vi "curr_measurement.vi"() -> ()   [LabVIEW 2018]
uses:
  <vilib>/Utility/file.llb/Write Delimited Spreadsheet (string).vi
  <instrlib>/Keithley 648X Series/Keithley 648X Series.lvlib
  <vilib>/Analysis/NI_AALBase.lvlib
panel:
  in  "Range (nA)":u16(ring)=6 items=["20mA", "2mA", "200uA", "20uA", "2uA", "200nA", "20nA", "2nA"]
  out "Waveform Graph":dbl[](graph)=[-9.351637e-09, -9.150208e-09, -1.001427e-08, -8.748215e-09, -8.522931e-09, -8.492725e-09, -9.785064e-09, -9.437517e-09, -9.272836e-09, -9.83262e-09, -9.335976e-09, -9.824586e-09, -9.370058e-09, -9.594313e-09, -9.258558e-09, -1.001164e-08, -9.479965e-09, -9.818684e-09, -8.33904e-09, -1.000336e-08, -9.407453e-09, -9.480965e-09, -9.881598e-09, -9.252624e-09, -9.527317e-09, -9.713401e-09, -8.709614e-09, -1.017135e-08, -9.863273e-09, -9.304885e-09, -1.037396e-08, -8.691322e-09, -9.202171e-09, -9.427193e-09, -9.452378e-09, -9.301955e-09, -9.93608e-09, -1.016247e-08, -9.657593e-09, -9.639637e-09, -9.532354e-09, -9.976174e-09, -9.564596e-09, -9.419945e-09, -9.793799e-09, -9.572672e-09, -9.966555e-09, -9.634946e-09, -9.932353e-09, -9.015443e-09, -9.172623e-09, -9.54698e-09, -9.282637e-09, -9.429553e-09, -1.039608e-08, -9.177771e-09, -9.569834e-09, -9.949303e-09, -9.517366e-09, -9.941039e-09, -9.143115e-09, -9.300412e-09, -9.838465e-09, -1.04458e-08, -8.665026e-09, -1.010992e-08, -9.321636e-09, -9.305311e-09, -9.199045e-09, -9.379991e-09, -1.014202e-08, -9.659195e-09, -1.016863e-08, -8.558392e-09, -8.893284e-09, -9.430091e-09, -1.035581e-08, -8.855966e-09, -9.206192e-09, -9.404848e-09, -9.820688e-09, -9.750344e-09, -9.513444e-09, -9.751563e-09, -1.025721e-08, -9.897644e-09, -9.474945e-09, -9.120714e-09, -9.959159e-09, -9.044635e-09, -9.964291e-09, -9.179353e-09, -9.380761e-09, -9.697832e-09, -9.19995e-09, -9.515208e-09, -9.913225e-09, -9.952196e-09, -9.35025e-09, -9.10259e-09, -9.434953e-09]
  out "Current Error":dbl=4.475602666243125e-11
  out "Current Mean":dbl=-9.525059320000003e-09 format="%e"
  out "Measurements":dbl[](array[numeric])=[-9.150208e-09, -1.001427e-08, -8.748215e-09, -8.522931e-09, -8.492725e-09, -9.785064e-09, -9.437517e-09, -9.272836e-09, -9.83262e-09, -9.335976e-09, -9.824586e-09, -9.370058e-09, -9.594313e-09, -9.258558e-09, -1.001164e-08, -9.479965e-09, -9.818684e-09, -8.33904e-09, -1.000336e-08, -9.407453e-09, -9.480965e-09, -9.881598e-09, -9.252624e-09, -9.527317e-09, -9.713401e-09, -8.709614e-09, -1.017135e-08, -9.863273e-09, -9.304885e-09, -1.037396e-08, -8.691322e-09, -9.202171e-09, -9.427193e-09, -9.452378e-09, -9.301955e-09, -9.93608e-09, -1.016247e-08, -9.657593e-09, -9.639637e-09, -9.532354e-09, -9.976174e-09, -9.564596e-09, -9.419945e-09, -9.793799e-09, -9.572672e-09, -9.966555e-09, -9.634946e-09, -9.932353e-09, -9.015443e-09, -9.172623e-09, -9.54698e-09, -9.282637e-09, -9.429553e-09, -1.039608e-08, -9.177771e-09, -9.569834e-09, -9.949303e-09, -9.517366e-09, -9.941039e-09, -9.143115e-09, -9.300412e-09, -9.838465e-09, -1.04458e-08, -8.665026e-09, -1.010992e-08, -9.321636e-09, -9.305311e-09, -9.199045e-09, -9.379991e-09, -1.014202e-08, -9.659195e-09, -1.016863e-08, -8.558392e-09, -8.893284e-09, -9.430091e-09, -1.035581e-08, -8.855966e-09, -9.206192e-09, -9.404848e-09, -9.820688e-09, -9.750344e-09, -9.513444e-09, -9.751563e-09, -1.025721e-08, -9.897644e-09, -9.474945e-09, -9.120714e-09, -9.959159e-09, -9.044635e-09, -9.964291e-09, -9.179353e-09, -9.380761e-09, -9.697832e-09, -9.19995e-09, -9.515208e-09, -9.913225e-09, -9.952196e-09, -9.35025e-09, -9.10259e-09, -9.434953e-09]
  out "error out":T1
  in  "Insert Voltage;Divider Current":string="3498.5;714.27"
  out "Stop Time string":string="20/02/2023 10:43:20"
  in  "file path (dialog if empty)":path=path "C:/Users/david/cernbox/Work/Detectors-Characterizations/monitoringGEM/P5_measurements/20022023/20022023.csv"
  out "Format Data":string[](array[string])=["Start time:", "Stop time:", "Voltage/Divider Current:", "Mean Anodic Current(A):", "Gaussian Error(A):"]
  out "Start time string":string="20/02/2023 10:42:43,00"
  in  "Interactions+1":i32=101
  out "Last measurement":dbl=-9.434953e-09
  in  "Autorange (T: Enable)":bool
  in  "error in (no error)":errorcluster
  in  "VISA resource name":refnum<visa-resource-name>="GPIB0::22::INSTR"
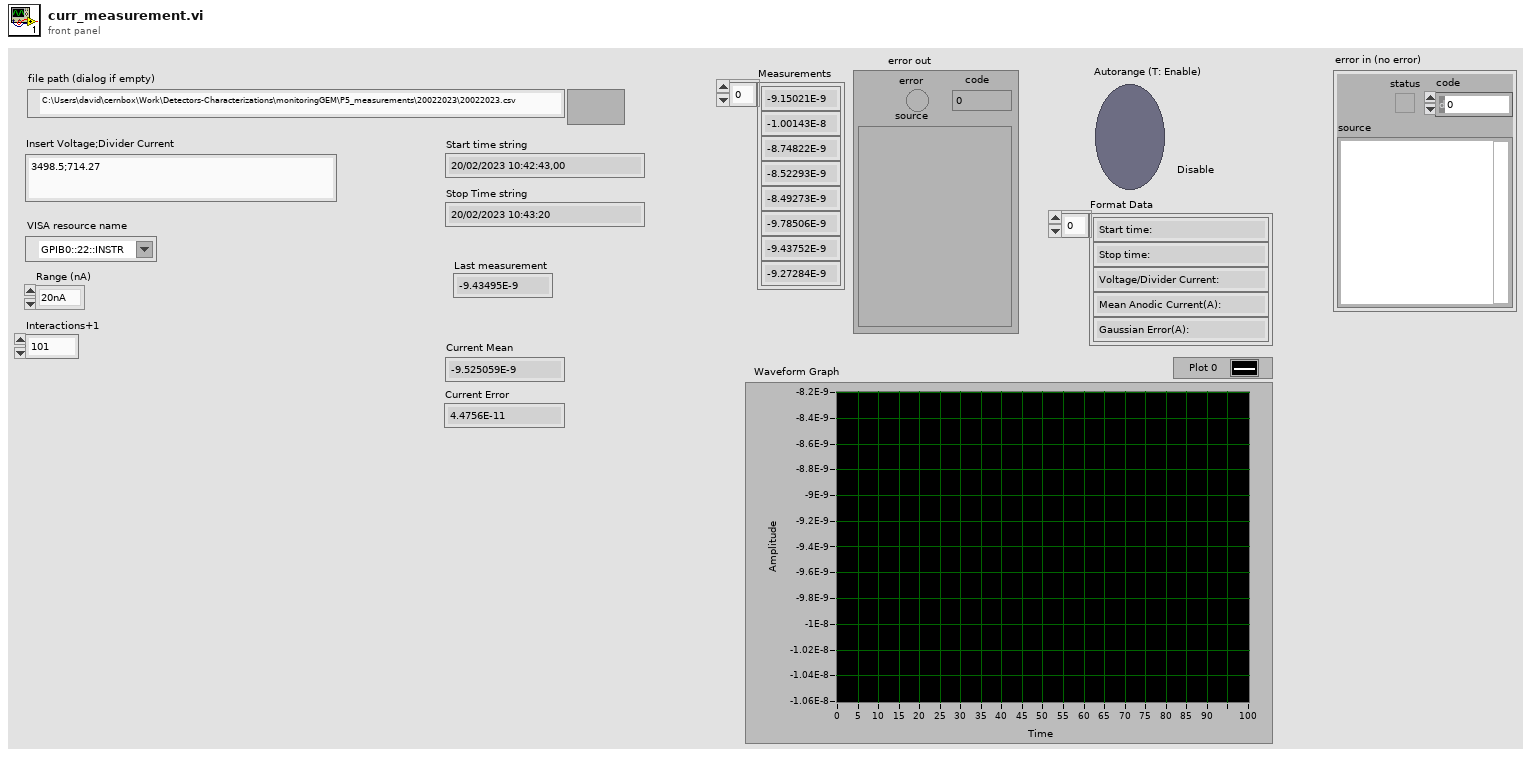
[diagram p1: front panel]
types:
  T1 = cluster{"error":bool, "code":i32, "source":string}
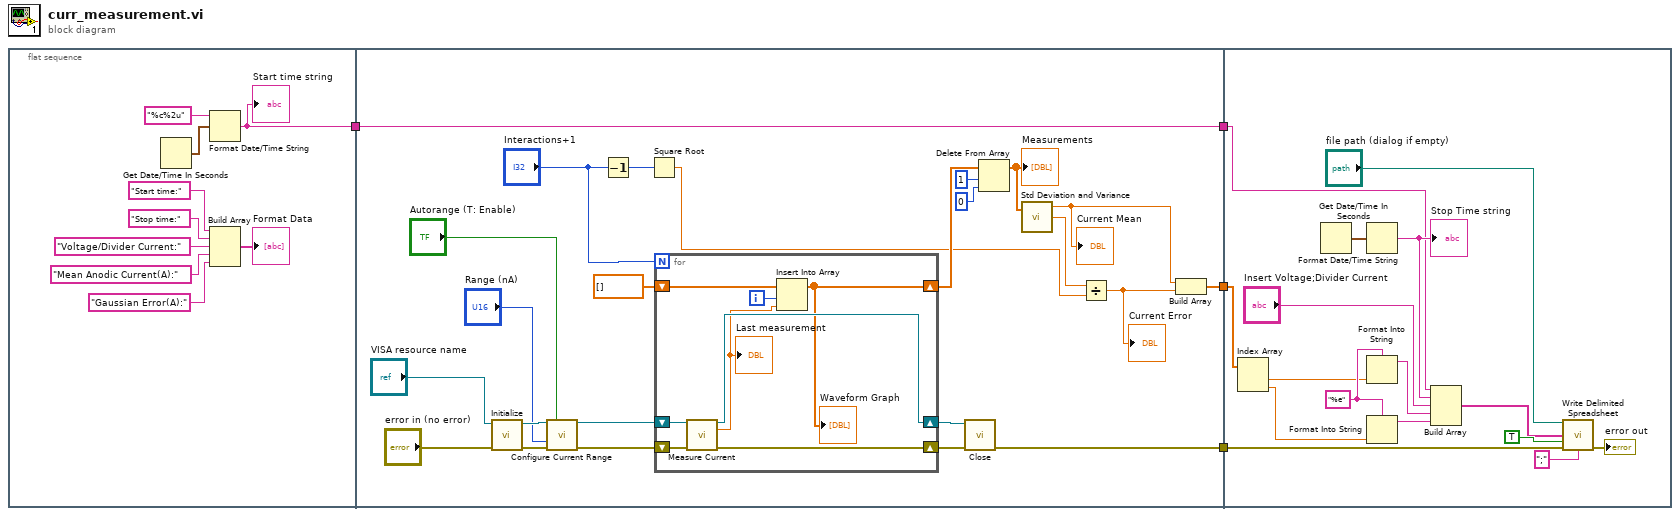
[diagram p0: block diagram]
diagram:
  n1 = flat-sequence {
    tunnel: [w5] -> w2
    tunnel: [w27] -> w4
    tunnel: [w18] -> w3
    tunnel: w2 -> [w18]
    tunnel: [w17] -> w1
    tunnel: w4 -> [w50]
    tunnel: w3 -> [w49]
    tunnel: w1 -> [w46]
    frame #0 {
      n2 = Get Date/Time In Seconds() -> (seconds since 1Jan1904=w13:timestamp)
      n3 = Format Date/Time String(time format string (%c)="%c%2u", seconds (now)=w13) -> (date/time string=w5:string)  [unwired: 1 in]
      "Start time string" <- w5
      n4 = Build Array("Start time:", "Stop time:", "Voltage/Divider Current:", "Mean Anodic Current(A):", "Gaussian Error(A):") -> (→"Format Data":string[])
    }
    frame #1 {
      n5 = call <instrlib>:"Initialize.vi"("error in (no error)"="error in (no error)", "VISA resource name"="VISA resource name") -> ("error out"=w34:errorcluster, "VISA resource name out"=w35:refnum<visa-resource-name>)  [unwired: 8 in]
      n6 = call <instrlib>:"Configure Current Range.vi"("VISA resource name"=w35, "Autorange (T: Enable)"="Autorange (T: Enable)", "Upper Measurement Range (200uA)"="Range (nA)", "error in (no error)"=w34) -> ("VISA resource name out"=w32:refnum<visa-resource-name>, "error out"=w31:errorcluster)  [unwired: 10 in]
      n7 = Decrement(x="Interactions+1") -> (x-1=w14:i32)
      n8 = Square Root(x=w14) -> (sqrt(x)=w22:dbl)
      n9 = for {
        N: "Interactions+1" -> [_]
        shift-right: [w43] -> w30
        shift-left: w32 -> [w45]
        shift-right: [w42] -> w29
        shift-left: w31 -> [w44]
        shift-right: [w38] -> w24
        shift-left: dbl[] [] ("array") -> [w41]
        i -> [w39]
        n10 = call <instrlib>:"Measure Current.vi"("VISA resource name"=w45, "error in (no error)"=w44) -> ("VISA resource name out"=w43:refnum<visa-resource-name>, "Measurement"=w40:dbl, "error out"=w42:errorcluster)  [unwired: 11 in]
        "Last measurement" <- w40
        n11 = Insert Into Array(array=w41, index=w39, new element=w40) -> (w38:dbl[])
        "Waveform Graph" <- w38
      }
      n12 = call <instrlib>:"Close.vi"("error in (no error)"=w29, "VISA resource name"=w30) -> ("error out"=w27:errorcluster)  [unwired: 9 in]
      n13 = Delete From Array(array=w24, length=1, index=0) -> (array with subset deleted=w23:dbl[])  [unwired: 1 out]
      "Measurements" <- w23
      n14 = call <vilib>:"Std Deviation and Variance.vi"("X"=w23) -> ("mean"=w20:dbl, "standard deviation"=w21:dbl)  [unwired: 1 in, 1 out]
      "Current Mean" <- w20
      n15 = Divide(x=w21, y=w22) -> (x/y=w19:dbl)
      "Current Error" <- w19
      n16 = Build Array(w20, w19) -> (w17:dbl[])
    }
    frame #2 {
      w52 = "%e" ("format (%.3f)")
      n17 = Index Array(array=w46) -> (element #1=w48:dbl, element #2=w47:dbl)  [unwired: 2 in]
      n18 = Get Date/Time In Seconds() -> (seconds since 1Jan1904=w61:timestamp)
      n19 = Format Date/Time String(seconds (now)=w61) -> (date/time string=w55:string)  [unwired: 2 in]
      "Stop Time string" <- w55
      n20 = Format Into String(format string=w52, w48) -> (resulting string=w59:string)  [unwired: 2 in, 1 out]
      n21 = Format Into String(format string=w52, w47) -> (resulting string=w58:string)  [unwired: 2 in, 1 out]
      n22 = Build Array(w49, w55, "Insert Voltage;Divider Current", w59, w58) -> (w57:string[])
      n23 = call-poly <vilib>:"Write Delimited Spreadsheet.vi"("file path (dialog if empty)"="file path (dialog if empty)", "1D data"=w57, "append to file? (new file:F)"=TRUE, "error in (no error)"=w50, "delimiter (\\t)"=";" ("delimiter (\\t)")) -> ("error out"=→"error out":errorcluster)  [unwired: 9 in, 1 out]
    }
  }
